vi "Dielectric vs Temperature Measurement (4263B).vi"() -> ()   [LabVIEW 2010]
uses:
  <vilib>/Instr/_visa.llb/VISA Configure Serial Port (Instr).vi
  Instance          14 22Saved   K vs T (4284A) .vi
  Instance          13 22Saved   K vs T (4284A) .vi
  Instance          12 22Saved   K vs T (4284A) .vi
  Instance          11 22Saved   K vs T (4284A) .vi
  Instance          26 22Saved   K vs T (4284A) .vi
  Instance          25 22Saved   K vs T (4284A) .vi
  Instance          10 22Saved   K vs T (4284A) .vi
  Instance           9 22Saved   K vs T (4284A) .vi
  Instance           8 22Saved   K vs T (4284A) .vi
  Instance           7 22Saved   K vs T (4284A) .vi
  Instance          24 22Saved   K vs T (4284A) .vi
  Instance          22 22Saved   K vs T (4284A) .vi
  Instance          20 22Saved   K vs T (4284A) .vi
  Instance          18 22Saved   K vs T (4284A) .vi
  Instance          23 22Saved   K vs T (4284A) .vi
  Instance          21 22Saved   K vs T (4284A) .vi
  Instance          19 22Saved   K vs T (4284A) .vi
  Instance          17 22Saved   K vs T (4284A) .vi
  Instance           6 22Saved   K vs T (4284A) .vi
  <vilib>/Utility/file.llb/Write To Spreadsheet File (DBL).vi
panel:
  in  "?":string="100"
  in  "?":string
  in  "?":string
  in  "?":string
  in  "tand100k":dbl[](array[numeric])
  in  "tand10k":dbl[](array[numeric])
  in  "tand1k":dbl[](array[numeric])
  in  "tand100":dbl[](array[numeric])
  in  "K100k":dbl[](array[numeric])
  in  "K10k":dbl[](array[numeric])
  in  "K1k":dbl[](array[numeric])
  in  "K100":dbl[](array[numeric])
  in  "Temp100k":dbl[](array[numeric])
  in  "Temp10k":dbl[](array[numeric])
  in  "Temp1k":dbl[](array[numeric])
  in  "Temp100":dbl[](array[numeric])
  out "Temp100kHz":dbl format="%#_3g"
  out "Temp10kHz":dbl format="%#_3g"
  out "tand100":dbl
  out "Temp1kHz":dbl format="%#_3g"
  in  "VISA Omega (Serial - COM6)":refnum<visa-resource-name>
  in  "VISA Agilent 4263B (GPIB)":refnum<visa-resource-name>
  in  "Run":bool
  out "Thickness":dbl
  out "Area":dbl
  in  "stop":bool
  out "tand100k":dbl
  out "tand10k":dbl
  out "tand1k":dbl
  out "K100k":dbl
  out "K10k":dbl
  out "K1k":dbl
  out "K100":dbl
  out "C100k":dbl
  out "C10k":dbl
  out "C1k":dbl
  out "C100":dbl
  out "Temp100Hz":dbl format="%#_3g"
  out "Dielectric Loss vs. Temperature":cluster{"Y":dbl[], "Y":dbl[]}[](graph)
  out "Relative Permittivity vs. Temperature":cluster{"Y":dbl[], "Y":dbl[]}[](graph)
  in  "Comment (Sample's Name, compositions, whatever you want,..)":string
  in  "Thickness (mm)":dbl
  in  "Diameter (mm)":dbl
  in  "Path & File Name (*.txt)":path
  # "Sample Details"
  # "Frequency (Hz)"
  # "Temperature (C)"
  # "Capacitance (F)"
  # "Relative Permittivity"
  # "Dielectric Loss"
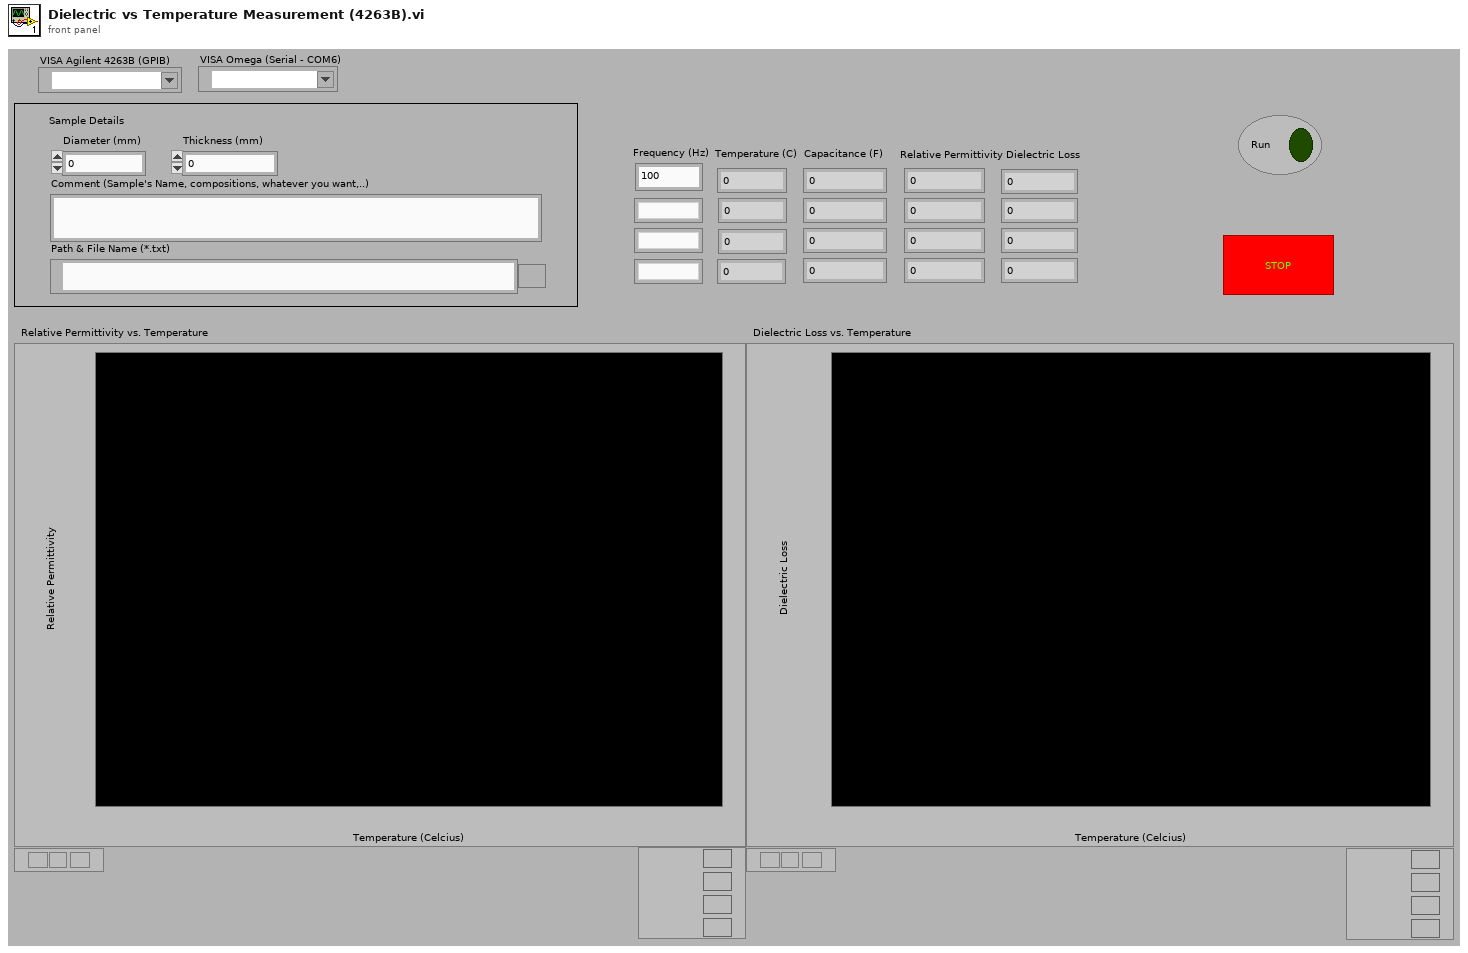
[diagram p1: front panel]
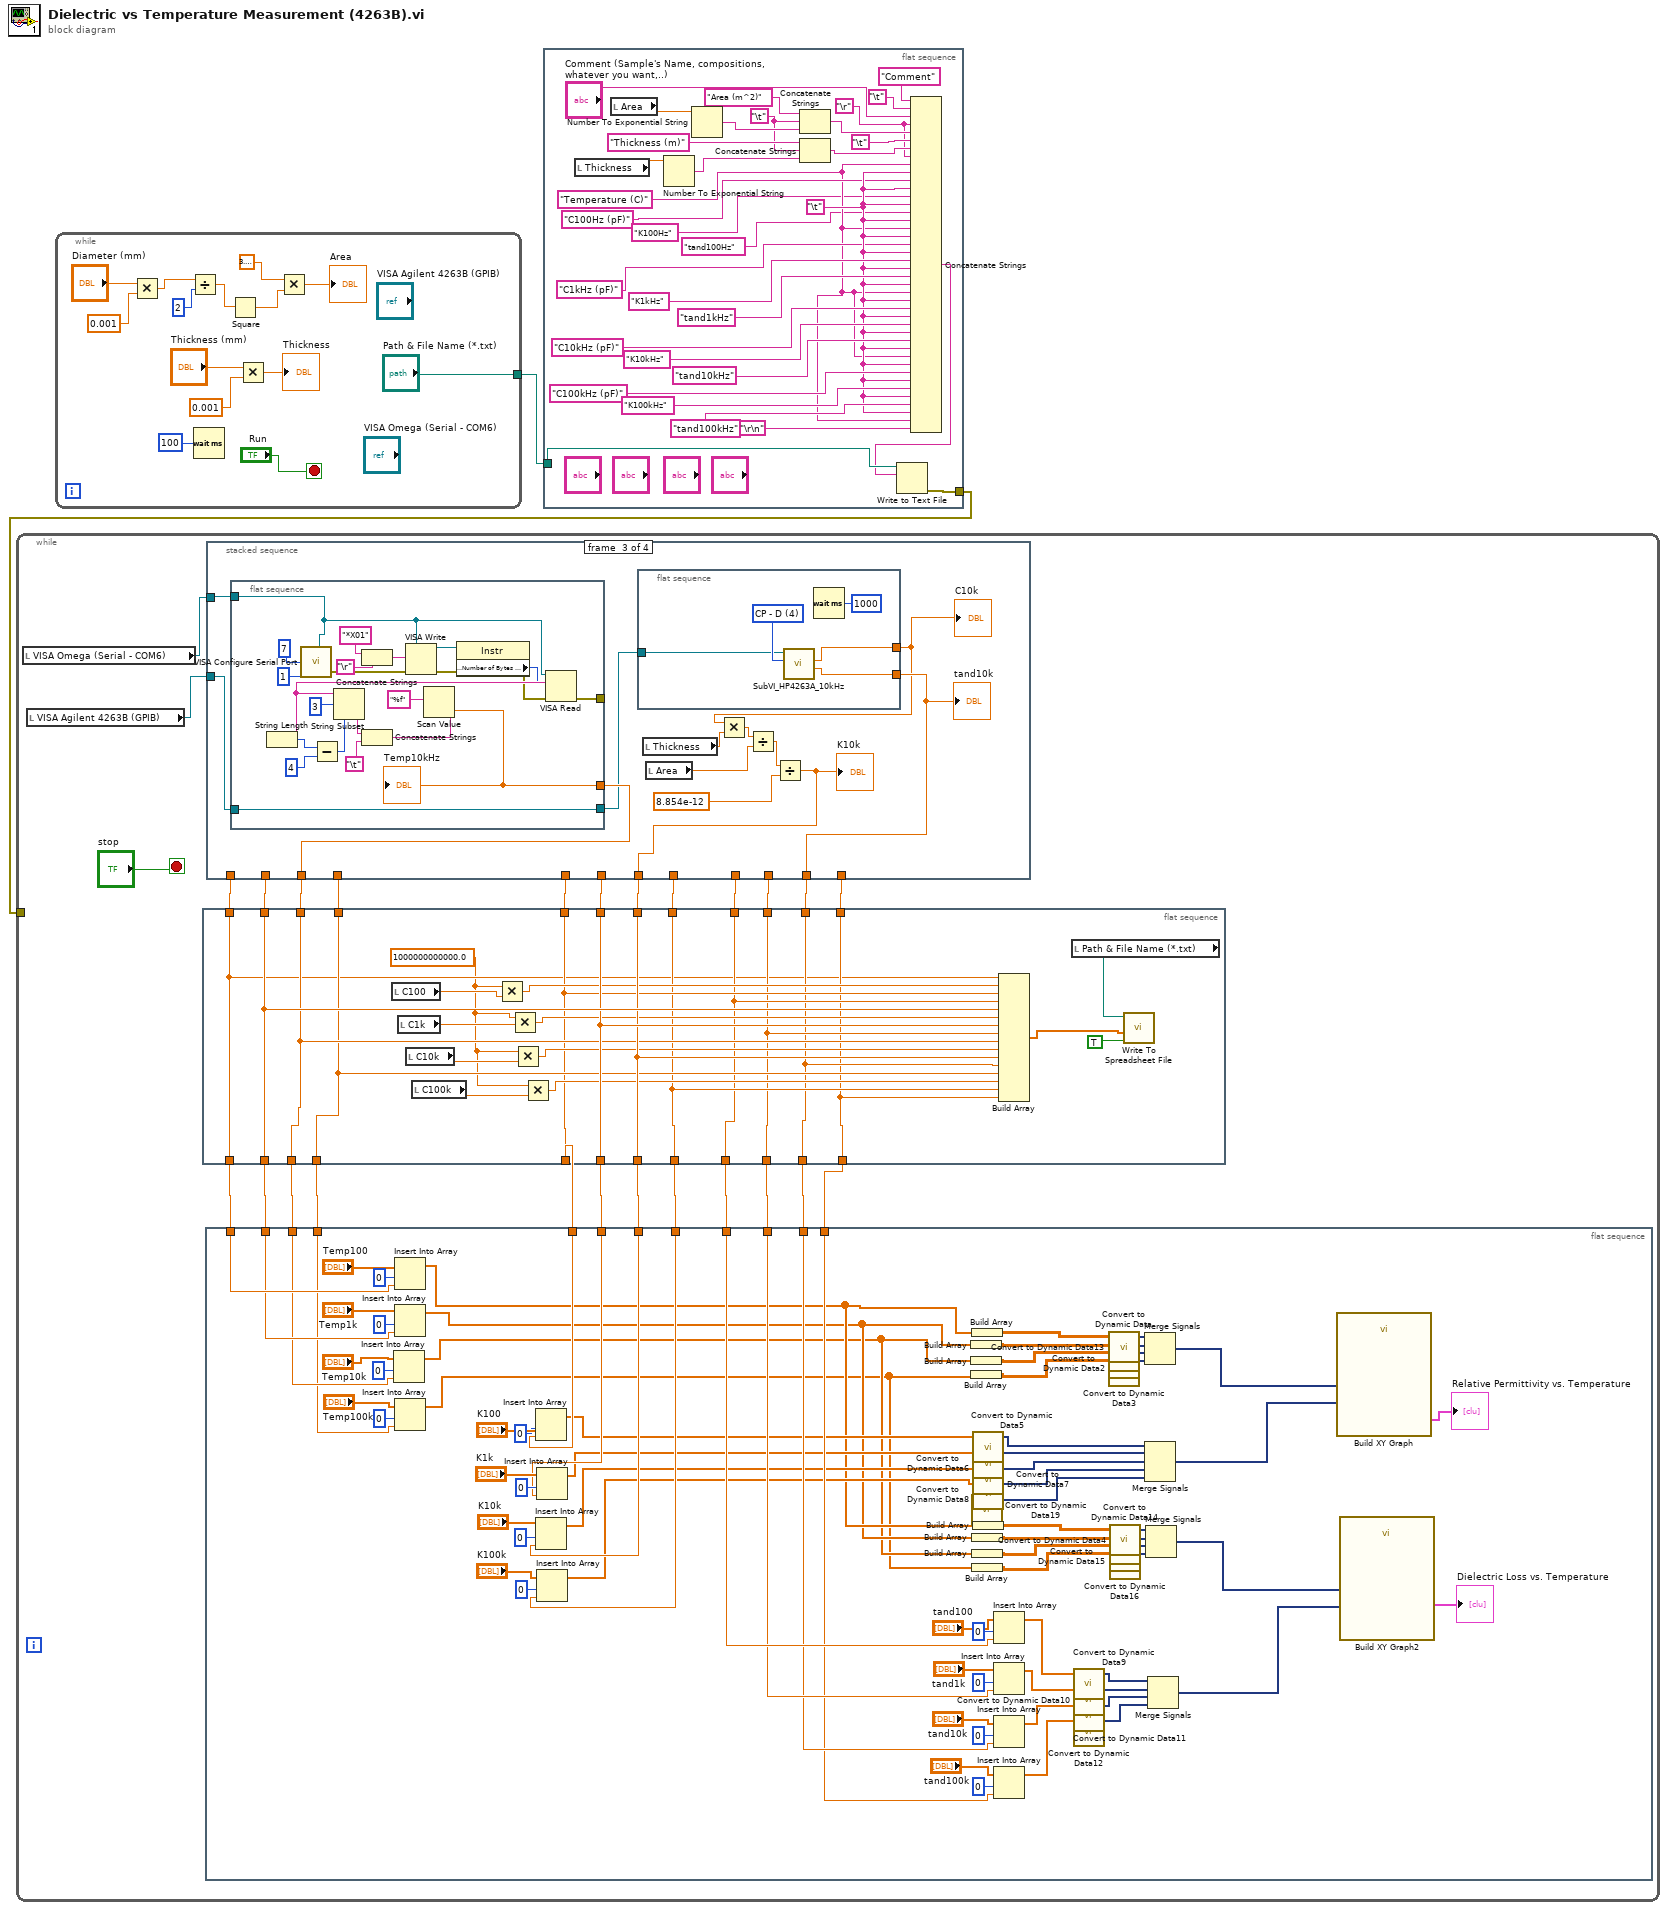
[diagram p0: block diagram]
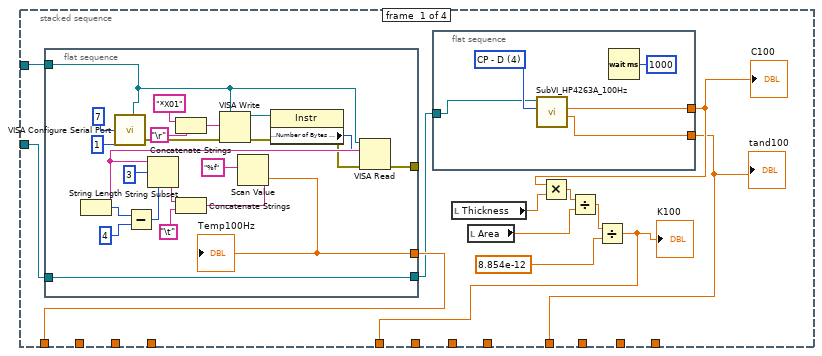
[diagram p2: hidden frame]
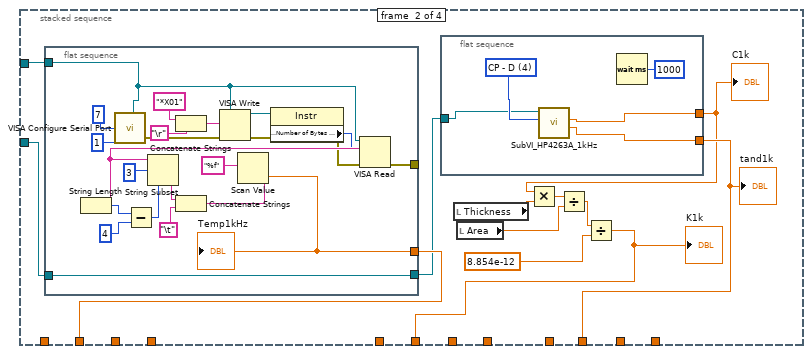
[diagram p3: hidden frame]
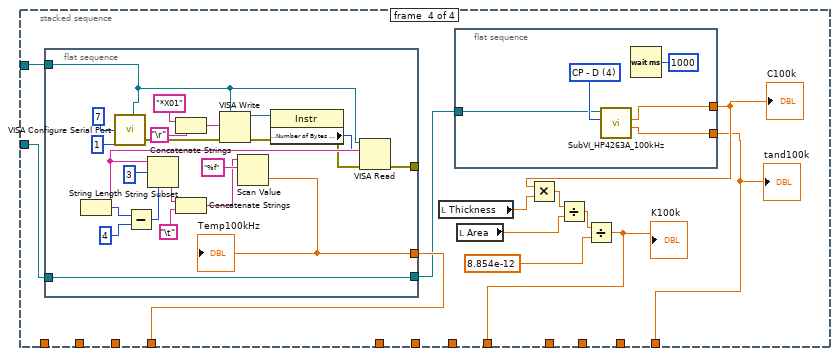
[diagram p4: hidden frame]
diagram:
  n1 = while {
    tunnel: w1 -> [_]
    stop <- "stop" stop-if-true
    n2 = local read "VISA Omega (Serial - COM6)"() -> (w16:refnum<visa-resource-name>)
    n3 = local read "VISA Agilent 4263B (GPIB)"() -> (w15:refnum<visa-resource-name>)
    n4 = flat-sequence {
      tunnel: w25 -> [w116]
      tunnel: w21 -> [w114]
      tunnel: w28 -> [w129]
      tunnel: w24 -> [w128]
      tunnel: w20 -> [w113]
      tunnel: w27 -> [w118]
      tunnel: w23 -> [w127]
      tunnel: w19 -> [w112]
      tunnel: w26 -> [w117]
      tunnel: w22 -> [w115]
      tunnel: w18 -> [w111]
      tunnel: [w129] -> w13
      tunnel: [w128] -> w9
      tunnel: [w127] -> w8
      tunnel: [w118] -> w12
      tunnel: [w117] -> w11
      tunnel: [w116] -> w10
      tunnel: [w115] -> w7
      tunnel: [w114] -> w6
      tunnel: [w113] -> w5
      tunnel: [w112] -> w4
      tunnel: [w111] -> w3
      tunnel: w17 -> [w110]
      tunnel: [w110] -> w14
      frame #0 {
        w109 = 1000000000000.0 ("x")
        n5 = local read "C100"() -> (w126:dbl)
        n6 = local read "C1k"() -> (w121:dbl)
        n7 = local read "C10k"() -> (w120:dbl)
        n8 = local read "C100k"() -> (w119:dbl)
        n9 = Multiply(x=w109, y=w126) -> (x*y=w125:dbl)
        n10 = Multiply(x=w109, y=w121) -> (x*y=w124:dbl)
        n11 = Multiply(x=w109, y=w120) -> (x*y=w123:dbl)
        n12 = Multiply(x=w109, y=w119) -> (x*y=w122:dbl)
        n13 = Build Array(w110, w125, w116, w114, w129, w124, w128, w113, w118, w123, w127, w112, w117, w122, w115, w111) -> (w132:dbl[])
        n14 = local read "Path & File Name (*.txt)"() -> (w130:path)
        n15 = call-poly <vilib>:"Write To Spreadsheet File.vi"("append to file? (new file:F)"=TRUE, "1D data"=w132, "file path (dialog if empty)"=w130) -> ()  [unwired: 5 in, 1 out]
      }
    }
    n16 = flat-sequence {
      tunnel: w14 -> [w75]
      tunnel: w13 -> [w74]
      tunnel: w12 -> [w73]
      tunnel: w11 -> [w72]
      tunnel: w10 -> [w71]
      tunnel: w9 -> [w70]
      tunnel: w8 -> [w69]
      tunnel: w7 -> [w68]
      tunnel: w6 -> [w67]
      tunnel: w5 -> [w66]
      tunnel: w4 -> [w65]
      tunnel: w3 -> [w64]
      frame #0 {
        n17 = Insert Into Array(array="Temp10k", index=0, new element=w73) -> (w35:dbl[])
        n18 = Insert Into Array(array="Temp100", index=0, new element=w75) -> (w37:dbl[])
        n19 = Insert Into Array(array="Temp1k", index=0, new element=w74) -> (w36:dbl[])
        n20 = Insert Into Array(array="Temp100k", index=0, new element=w72) -> (w34:dbl[])
        n21 = Insert Into Array(array="K100", index=0, new element=w71) -> (w57:dbl[])
        n22 = Insert Into Array(array="K10k", index=0, new element=w69) -> (w55:dbl[])
        n23 = Insert Into Array(array="K1k", index=0, new element=w70) -> (w56:dbl[])
        n24 = Insert Into Array(array="K100k", index=0, new element=w68) -> (w54:dbl[])
        n25 = Build Array(w36) -> (w51:dbl[][])
        n26 = Build Array(w35) -> (w49:dbl[][])
        n27 = Build Array(w34) -> (w47:dbl[][])
        n28 = Build Array(w37) -> (w53:dbl[][])
        n29 = call "Convert to Dynamic Data19"() -> ("Dynamic Data Type"=w31:dynamicdata)  [unwired: 4 in]
        n30 = Build Array(w36) -> (w40:dbl[][])
        n31 = Build Array(w35) -> (w42:dbl[][])
        n32 = Build Array(w34) -> (w44:dbl[][])
        n33 = call "Convert to Dynamic Data5"("Array"=w57) -> ("Dynamic Data Type"=w63:dynamicdata)  [unwired: 3 in]
        n34 = call "Convert to Dynamic Data6"("Array"=w56) -> ("Dynamic Data Type"=w62:dynamicdata)  [unwired: 3 in]
        n35 = call "Convert to Dynamic Data7"("Array"=w55) -> ("Dynamic Data Type"=w61:dynamicdata)  [unwired: 3 in]
        n36 = call "Convert to Dynamic Data8"("Array"=w54) -> ("Dynamic Data Type"=w60:dynamicdata)  [unwired: 3 in]
        n37 = Build Array(w37) -> (w38:dbl[][])
        n38 = Insert Into Array(array="tand100", index=0, new element=w67) -> (w93:dbl[])
        n39 = Insert Into Array(array="tand1k", index=0, new element=w66) -> (w94:dbl[])
        n40 = Insert Into Array(array="tand10k", index=0, new element=w65) -> (w95:dbl[])
        n41 = Insert Into Array(array="tand100k", index=0, new element=w64) -> (w96:dbl[])
        n42 = call "Convert to Dynamic Data9"("Array"=w93) -> ("Dynamic Data Type"=w78:dynamicdata)  [unwired: 3 in]
        n43 = call "Convert to Dynamic Data10"("Array"=w94) -> ("Dynamic Data Type"=w79:dynamicdata)  [unwired: 3 in]
        n44 = call "Convert to Dynamic Data11"("Array"=w95) -> ("Dynamic Data Type"=w32:dynamicdata)  [unwired: 3 in]
        n45 = call "Convert to Dynamic Data12"("Array"=w96) -> ("Dynamic Data Type"=w30:dynamicdata)  [unwired: 3 in]
        n46 = call "Convert to Dynamic Data13"("2D Array"=w53) -> ("Dynamic Data Type"=w52:dynamicdata)  [unwired: 3 in]
        n47 = call "Convert to Dynamic Data"("2D Array"=w51) -> ("Dynamic Data Type"=w50:dynamicdata)  [unwired: 3 in]
        n48 = call "Convert to Dynamic Data2"("2D Array"=w49) -> ("Dynamic Data Type"=w48:dynamicdata)  [unwired: 3 in]
        n49 = call "Convert to Dynamic Data3"("2D Array"=w47) -> ("Dynamic Data Type"=w46:dynamicdata)  [unwired: 3 in]
        n50 = call "Convert to Dynamic Data4"("2D Array"=w38) -> ("Dynamic Data Type"=w39:dynamicdata)  [unwired: 3 in]
        n51 = call "Convert to Dynamic Data14"("2D Array"=w40) -> ("Dynamic Data Type"=w41:dynamicdata)  [unwired: 3 in]
        n52 = call "Convert to Dynamic Data15"("2D Array"=w42) -> ("Dynamic Data Type"=w43:dynamicdata)  [unwired: 3 in]
        n53 = call "Convert to Dynamic Data16"("2D Array"=w44) -> ("Dynamic Data Type"=w45:dynamicdata)  [unwired: 3 in]
        n54 = Merge Signals(w52, w50, w48, w46) -> (w58:dynamicdata)
        n55 = Merge Signals(w63, w62, w61, w60, w31) -> (w59:dynamicdata)
        n56 = Merge Signals(w39, w41, w43, w45) -> (w33:dynamicdata)
        n57 = Merge Signals(w78, w79, w32, w30) -> (w80:dynamicdata)
        n58 = call "Build XY Graph"("Y Input"=w59, "X Input"=w58) -> ("XY Graph"=→"Relative Permittivity vs. Temperature":cluster{"Y":dbl[], "Y":dbl[]}[])  [unwired: 8 in, 1 out]
        n59 = call "Build XY Graph2"("Y Input"=w80, "X Input"=w33) -> ("XY Graph"=→"Dielectric Loss vs. Temperature":cluster{"Y":dbl[], "Y":dbl[]}[])  [unwired: 8 in, 1 out]
      }
    }
    n60 = stacked-sequence {
      tunnel: w16 -> [w144 w184 w224 w264]
      tunnel: w15 -> [w143 w183 w223 w263]
      tunnel: [w137 _ _ _] -> w17
      tunnel: [_ w177 _ _] -> w28
      tunnel: [_ _ w217 _] -> w27
      tunnel: [_ _ _ w257] -> w26
      tunnel: [w133 _ _ _] -> w25
      tunnel: [_ w176 _ _] -> w24
      tunnel: [_ _ w216 _] -> w23
      tunnel: [_ _ _ w256] -> w22
      tunnel: [w134 _ _ _] -> w21
      tunnel: [_ w175 _ _] -> w20
      tunnel: [_ _ w214 _] -> w19
      tunnel: [_ _ _ w253] -> w18
      frame #0 {
        n61 = flat-sequence {
          tunnel: w144 -> [w153]
          tunnel: [w152] -> _
          tunnel: [w151] -> w137
          tunnel: w143 -> [w150]
          tunnel: [w150] -> w136
          frame #0 {
            n62 = call-poly "VISA Configure Serial Port"("VISA resource name"=w153, "data bits (8)"=7, "parity (0:none)"=1) -> ("error out"=w158:errorcluster)  [unwired: 11 in, 1 out]
            n63 = Concatenate Strings("*X01", "\r") -> (w161:string)
            n64 = VISA Write(VISA resource name=w153, write buffer=w161, error in (no error)=w158) -> (VISA resource name out=w172:refnum<visa-resource-name>, error out=w162:errorcluster)  [unwired: 1 out]
            n65 = property class="Instr"(reference=w172, error in=w162) -> (error out=w163:errorcluster, "Serial Settings:Number of Bytes at Serial Port"=w164:u32)  [unwired: 1 out]
            n66 = VISA Read(VISA resource name=w153, byte count=w164, error in (no error)=w163) -> (read buffer=w165:string, error out=w152:errorcluster)  [unwired: 2 out]
            n67 = String Length(string=w165) -> (length=w167:i32)
            n68 = Subtract(x=w167, y=4) -> (x-y=w169:i32)
            n69 = String Subset(string=w165, offset (0)=3, length (rest)=w169) -> (substring=w170:string)
            n70 = Concatenate Strings(w170, "\t") -> (w154:string)
            n71 = Scan Value(string=w154, format string="%f") -> (value=w151:dbl)  [unwired: 1 in, 1 out]
            "Temp100Hz" <- w151
          }
        }
        n72 = flat-sequence {
          tunnel: w136 -> [w145]
          tunnel: [w147] -> w134
          tunnel: [w148] -> w135
          frame #0 {
            w146 = u16 4 items=["Z - Angle", "R - X", "Y - Angle", "G - B", "CP - D", "CP - Q", "CP - G", "CS - D", "CS - Q", "CS - RS", "LP - D", "LP - Q", "LP - G", "LS - D", "LS - Q", "LS - RS", "LS - DCR (option 001 only)", "LP - DCR (option 001 only)", "L2 - N (option 001 only)", "L2 - M (option 001 only)", "L2 - R2 (option 001 only)"] ("function (Z - Angle:0)")
            n73 = call "SubVI_HP4263A_100Hz.vi"("function (Z - Angle:0)"=w146, "VISA resource name"=w145) -> ("secondary reading"=w147:dbl, "primary reading"=w148:dbl)  [unwired: 2 in, 2 out]
            n74 = Wait (ms)(milliseconds to wait=u32 1000) -> ()  [unwired: 1 out]
          }
        }
        n75 = local read "Thickness"() -> (w142:dbl)
        n76 = local read "Area"() -> (w140:dbl)
        n77 = Multiply(x=w135, y=w142) -> (x*y=w141:dbl)
        n78 = Divide(x=w141, y=w140) -> (x/y=w139:dbl)
        n79 = Divide(x=w139, y=8.854e-12) -> (x/y=w133:dbl)
        "K100" <- w133
        "C100" <- w135
        "tand100" <- w134
      }
      frame #1 {
        n80 = flat-sequence {
          tunnel: w184 -> [w193]
          tunnel: [w192] -> _
          tunnel: [w191] -> w177
          tunnel: w183 -> [w190]
          tunnel: [w190] -> w173
          frame #0 {
            n81 = call-poly "VISA Configure Serial Port"("VISA resource name"=w193, "data bits (8)"=7, "parity (0:none)"=1) -> ("error out"=w198:errorcluster)  [unwired: 11 in, 1 out]
            n82 = Concatenate Strings("*X01", "\r") -> (w201:string)
            n83 = VISA Write(VISA resource name=w193, write buffer=w201, error in (no error)=w198) -> (VISA resource name out=w212:refnum<visa-resource-name>, error out=w202:errorcluster)  [unwired: 1 out]
            n84 = property class="Instr"(reference=w212, error in=w202) -> (error out=w203:errorcluster, "Serial Settings:Number of Bytes at Serial Port"=w204:u32)  [unwired: 1 out]
            n85 = VISA Read(VISA resource name=w193, byte count=w204, error in (no error)=w203) -> (read buffer=w205:string, error out=w192:errorcluster)  [unwired: 2 out]
            n86 = String Length(string=w205) -> (length=w207:i32)
            n87 = Subtract(x=w207, y=4) -> (x-y=w209:i32)
            n88 = String Subset(string=w205, offset (0)=3, length (rest)=w209) -> (substring=w210:string)
            n89 = Concatenate Strings(w210, "\t") -> (w194:string)
            n90 = Scan Value(string=w194, format string="%f") -> (value=w191:dbl)  [unwired: 1 in, 1 out]
            "Temp1kHz" <- w191
          }
        }
        n91 = flat-sequence {
          tunnel: w173 -> [w185]
          tunnel: [w187] -> w175
          tunnel: [w188] -> w174
          frame #0 {
            w186 = u16 4 items=["Z - Angle", "R - X", "Y - Angle", "G - B", "CP - D", "CP - Q", "CP - G", "CS - D", "CS - Q", "CS - RS", "LP - D", "LP - Q", "LP - G", "LS - D", "LS - Q", "LS - RS", "LS - DCR (option 001 only)", "LP - DCR (option 001 only)", "L2 - N (option 001 only)", "L2 - M (option 001 only)", "L2 - R2 (option 001 only)"] ("function (Z - Angle:0)")
            n92 = call "SubVI_HP4263A_1kHz.vi"("function (Z - Angle:0)"=w186, "VISA resource name"=w185) -> ("secondary reading"=w187:dbl, "primary reading"=w188:dbl)  [unwired: 2 in, 2 out]
            n93 = Wait (ms)(milliseconds to wait=u32 1000) -> ()  [unwired: 1 out]
          }
        }
        n94 = local read "Thickness"() -> (w182:dbl)
        n95 = local read "Area"() -> (w180:dbl)
        n96 = Multiply(x=w174, y=w182) -> (x*y=w181:dbl)
        n97 = Divide(x=w181, y=w180) -> (x/y=w179:dbl)
        n98 = Divide(x=w179, y=8.854e-12) -> (x/y=w176:dbl)
        "K1k" <- w176
        "tand1k" <- w175
        "C1k" <- w174
      }
      frame #2 {
        n99 = flat-sequence {
          tunnel: w224 -> [w233]
          tunnel: [w232] -> _
          tunnel: [w231] -> w217
          tunnel: w223 -> [w230]
          tunnel: [w230] -> w215
          frame #0 {
            n100 = call-poly "VISA Configure Serial Port"("VISA resource name"=w233, "data bits (8)"=7, "parity (0:none)"=1) -> ("error out"=w238:errorcluster)  [unwired: 11 in, 1 out]
            n101 = Concatenate Strings("*X01", "\r") -> (w241:string)
            n102 = VISA Write(VISA resource name=w233, write buffer=w241, error in (no error)=w238) -> (VISA resource name out=w252:refnum<visa-resource-name>, error out=w242:errorcluster)  [unwired: 1 out]
            n103 = property class="Instr"(reference=w252, error in=w242) -> (error out=w243:errorcluster, "Serial Settings:Number of Bytes at Serial Port"=w244:u32)  [unwired: 1 out]
            n104 = VISA Read(VISA resource name=w233, byte count=w244, error in (no error)=w243) -> (read buffer=w245:string, error out=w232:errorcluster)  [unwired: 2 out]
            n105 = String Length(string=w245) -> (length=w247:i32)
            n106 = Subtract(x=w247, y=4) -> (x-y=w249:i32)
            n107 = String Subset(string=w245, offset (0)=3, length (rest)=w249) -> (substring=w250:string)
            n108 = Concatenate Strings(w250, "\t") -> (w234:string)
            n109 = Scan Value(string=w234, format string="%f") -> (value=w231:dbl)  [unwired: 1 in, 1 out]
            "Temp10kHz" <- w231
          }
        }
        n110 = flat-sequence {
          tunnel: w215 -> [w225]
          tunnel: [w226] -> w214
          tunnel: [w227] -> w213
          frame #0 {
            w228 = u16 4 items=["Z - Angle", "R - X", "Y - Angle", "G - B", "CP - D", "CP - Q", "CP - G", "CS - D", "CS - Q", "CS - RS", "LP - D", "LP - Q", "LP - G", "LS - D", "LS - Q", "LS - RS", "LS - DCR (option 001 only)", "LP - DCR (option 001 only)", "L2 - N (option 001 only)", "L2 - M (option 001 only)", "L2 - R2 (option 001 only)"] ("function (Z - Angle:0)")
            n111 = call "SubVI_HP4263A_10kHz.vi"("function (Z - Angle:0)"=w228, "VISA resource name"=w225) -> ("secondary reading"=w226:dbl, "primary reading"=w227:dbl)  [unwired: 2 in, 2 out]
            n112 = Wait (ms)(milliseconds to wait=u32 1000) -> ()  [unwired: 1 out]
          }
        }
        n113 = local read "Thickness"() -> (w222:dbl)
        n114 = local read "Area"() -> (w220:dbl)
        n115 = Multiply(x=w213, y=w222) -> (x*y=w221:dbl)
        n116 = Divide(x=w221, y=w220) -> (x/y=w219:dbl)
        n117 = Divide(x=w219, y=8.854e-12) -> (x/y=w216:dbl)
        "K10k" <- w216
        "C10k" <- w213
        "tand10k" <- w214
      }
      frame #3 {
        n118 = flat-sequence {
          tunnel: w264 -> [w274]
          tunnel: [w273] -> _
          tunnel: [w272] -> w257
          tunnel: w263 -> [w271]
          tunnel: [w271] -> w255
          frame #0 {
            n119 = call-poly "VISA Configure Serial Port"("VISA resource name"=w274, "data bits (8)"=7, "parity (0:none)"=1) -> ("error out"=w278:errorcluster)  [unwired: 11 in, 1 out]
            n120 = Concatenate Strings("*X01", "\r") -> (w281:string)
            n121 = VISA Write(VISA resource name=w274, write buffer=w281, error in (no error)=w278) -> (VISA resource name out=w292:refnum<visa-resource-name>, error out=w282:errorcluster)  [unwired: 1 out]
            n122 = property class="Instr"(reference=w292, error in=w282) -> (error out=w283:errorcluster, "Serial Settings:Number of Bytes at Serial Port"=w284:u32)  [unwired: 1 out]
            n123 = VISA Read(VISA resource name=w274, byte count=w284, error in (no error)=w283) -> (read buffer=w285:string, error out=w273:errorcluster)  [unwired: 2 out]
            n124 = String Length(string=w285) -> (length=w287:i32)
            n125 = Subtract(x=w287, y=4) -> (x-y=w289:i32)
            n126 = String Subset(string=w285, offset (0)=3, length (rest)=w289) -> (substring=w290:string)
            n127 = Concatenate Strings(w290, "\t") -> (w270:string)
            n128 = Scan Value(string=w270, format string="%f") -> (value=w272:dbl)  [unwired: 1 in, 1 out]
            "Temp100kHz" <- w272
          }
        }
        n129 = local read "Thickness"() -> (w262:dbl)
        n130 = flat-sequence {
          tunnel: w255 -> [w265]
          tunnel: [w266] -> w253
          tunnel: [w267] -> w254
          frame #0 {
            w268 = u16 4 items=["Z - Angle", "R - X", "Y - Angle", "G - B", "CP - D", "CP - Q", "CP - G", "CS - D", "CS - Q", "CS - RS", "LP - D", "LP - Q", "LP - G", "LS - D", "LS - Q", "LS - RS", "LS - DCR (option 001 only)", "LP - DCR (option 001 only)", "L2 - N (option 001 only)", "L2 - M (option 001 only)", "L2 - R2 (option 001 only)"] ("function (Z - Angle:0)")
            n131 = call "SubVI_HP4263A_100kHz.vi"("function (Z - Angle:0)"=w268, "VISA resource name"=w265) -> ("secondary reading"=w266:dbl, "primary reading"=w267:dbl)  [unwired: 2 in, 2 out]
            n132 = Wait (ms)(milliseconds to wait=u32 1000) -> ()  [unwired: 1 out]
          }
        }
        n133 = local read "Area"() -> (w260:dbl)
        n134 = Multiply(x=w254, y=w262) -> (x*y=w261:dbl)
        n135 = Divide(x=w261, y=w260) -> (x/y=w259:dbl)
        n136 = Divide(x=w259, y=8.854e-12) -> (x/y=w256:dbl)
        "K100k" <- w256
        "C100k" <- w254
        "tand100k" <- w253
      }
    }
  }
  n137 = while {
    tunnel: ["Path & File Name (*.txt)"] -> w2
    stop <- "Run" stop-if-true
    n138 = Multiply(x="Diameter (mm)", y=0.001) -> (x*y=w301:dbl)
    n139 = Divide(x=w301, y=2) -> (x/y=w296:dbl)
    n140 = Wait (ms)(milliseconds to wait=u32 100) -> ()  [unwired: 1 out]
    n141 = Square(x=w296) -> (x^2=w297:dbl)
    n142 = Multiply(x="Thickness (mm)", y=0.001) -> (x*y=→"Thickness":dbl)
    n143 = Multiply(x=3.141592653589793, y=w297) -> (x*y=→"Area":dbl)
  }
  n144 = flat-sequence {
    tunnel: w2 -> [w333]
    tunnel: [w331] -> w1
    frame #0 {
      w313 = "\r"
      w315 = "\t"
      w309 = "Temperature (C)" ("string")
      w312 = "\t"
      n145 = local read "Thickness"() -> (w337:dbl)
      n146 = local read "Area"() -> (w338:dbl)
      n147 = Number To Exponential String(number=w337) -> (E-format string=w329:string)  [unwired: 3 in]
      n148 = Number To Exponential String(number=w338) -> (E-format string=w330:string)  [unwired: 3 in]
      n149 = Concatenate Strings("Area (m^2)" ("string"), w312, w330) -> (w334:string)
      n150 = Concatenate Strings("Thickness (m)" ("string"), w312, w329) -> (w328:string)
      n151 = Concatenate Strings("Comment" ("string"), "\t", "Comment (Sample's Name, compositions, whatever you want,..)", w313, w334, "\t", w328, w313, w309, w315, "C100Hz (pF)" ("string"), w315, "K100Hz" ("string"), w315, "tand100Hz" ("string"), w315, w309, w315, "C1kHz (pF)" ("string"), w315, "K1kHz" ("string"), w315, "tand1kHz" ("string"), w315, w309, w315, "C10kHz (pF)" ("string"), w315, "K10kHz" ("string"), w315, "tand10kHz" ("string"), w315, w309, w315, "C100kHz (pF)" ("string"), w315, "K100kHz" ("string"), w315, "tand100kHz" ("string"), w315, w309, "\r\n") -> (w332:string)
      n152 = Write to Text File(file (use dialog)=w333, text=w332) -> (error out=w331:errorcluster)  [unwired: 2 in, 2 out]
    }
  }
